vi "ErrorDataReceived.vi"(4 "User Parameter":refnum<user-event>[](array[refnum]), 5 "Event Data":cluster{"sender":refnum<k24>, "e":refnum<k24>}, 6 "Control Ref":refnum<k24>, 7 "Event Common Data":T1) -> ()   [LabVIEW 2018, in "callback-system-exec.lvlib"]
uses:
  callback-system-exec.lvlib
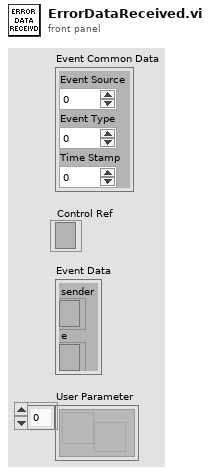
[diagram p1: front panel]
types:
  T1 = cluster{"Event Source":i32, "Event Type":u32, "Time Stamp":u32}
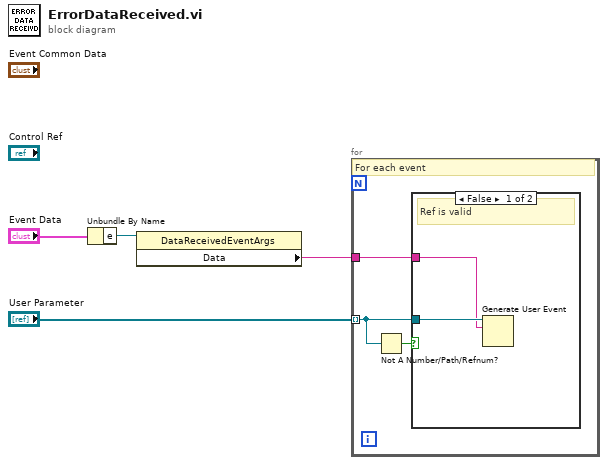
[diagram p0: block diagram]
diagram:
  n1 = Unbundle By Name("Event Data") -> ("e"=w3:refnum<k24>)
  n2 = property class="DataReceivedEventArgs"(reference=w3) -> ("Data"=w4:string)  [unwired: 1 in, 2 out]
  n3 = for {
    tunnel: "User Parameter" -> [w5] mode=indexing
    tunnel: w4 -> [w6]
    # "For each event"
    n4 = Not A Number/Path/Refnum?(number/path/refnum=w5) -> (NaN/Path/Refnum?=w7:bool)
    n5 = case shown="False" w7 {
      tunnel: w6 -> [w8 _]
      tunnel: w5 -> [w9 _]
      frame False {
        # "Ref is valid"
        n6 = Generate User Event(user event=w9, event data cluster=w8) -> ()  [unwired: 2 in, 2 out]
      }
      frame True {
      }
    }
  }
